vi "Unzip-Mercury-iXX.vi"(8 "error in (no error)":errorcluster) -> (0 "error out":errorcluster)   [LabVIEW 2019]
uses:
  <userlib>/_OpenG.lib/string/string.llb/Trim Whitespace (String)__ogtk.vi
  <vilib>/zip/NI_Unzip.lvlib
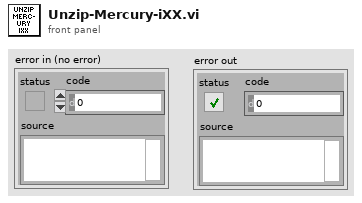
[diagram p1: front panel]
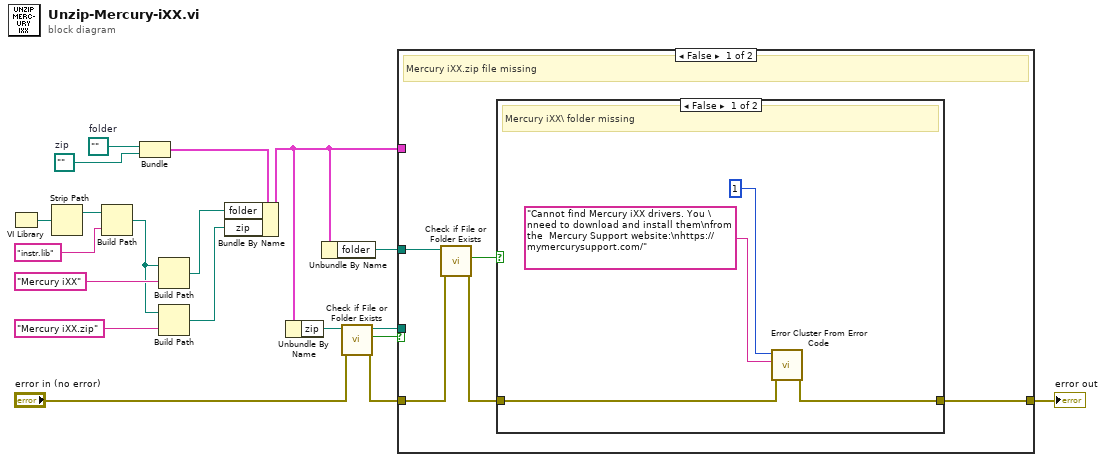
[diagram p0: block diagram]
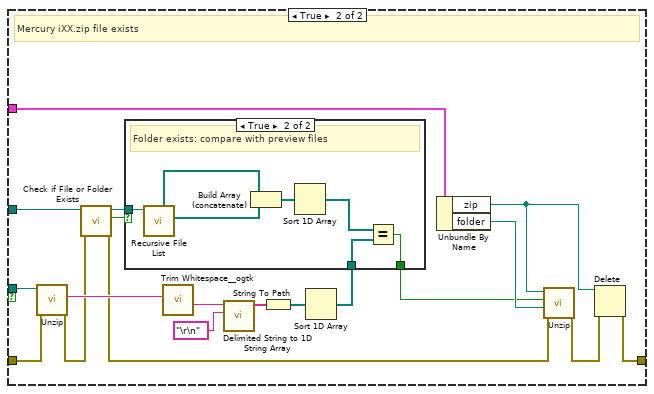
[diagram p3: hidden frame]
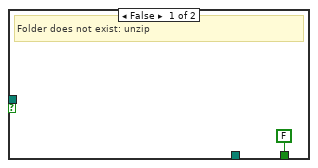
[diagram p4: hidden frame]
diagram:
  w13 = path ""  # zip
  w14 = path ""  # folder
  n1 = VI Library() -> (path=w19:path)
  n2 = Strip Path(path=w19) -> (stripped path=w18:path)  [unwired: 1 out]
  n3 = Build Path(base path=w18, name or relative path="instr.lib") -> (appended path=w15:path)
  n4 = Bundle("folder"=w14, "zip"=w13) -> (w12:cluster{"folder":path, "zip":path})  [unwired: 1 in]
  n5 = Build Path(base path=w15, name or relative path="Mercury iXX") -> (appended path=w11:path)
  n6 = Build Path(base path=w15, name or relative path="Mercury iXX.zip") -> (appended path=w10:path)
  n7 = Bundle By Name(cluster=w12, "folder"=w11, "zip"=w10) -> (w5:cluster{"folder":path, "zip":path})
  n8 = Unbundle By Name(w5) -> ("zip"=w9:path)
  n9 = Unbundle By Name(w5) -> ("folder"=w6:path)
  n10 = call <vilib>:"Check if File or Folder Exists.vi"("error in (no error)"="error in (no error)", "path"=w9) -> ("error out"=w3:errorcluster, "file or folder exists?"=w2:bool, "dup path"=w4:path)  [unwired: 7 in]
  n11 = case shown="False" w2 {
    tunnel: [w20 w48] -> w8
    tunnel: w6 -> [w24 w47]
    tunnel: w5 -> [_ w46]
    tunnel: w4 -> [_ w39]
    tunnel: w3 -> [w23 w37]
    frame False {
      # "Mercury iXX.zip file missing"
      n12 = call <vilib>:"Check if File or Folder Exists.vi"("error in (no error)"=w23, "path"=w24) -> ("error out"=w21:errorcluster, "file or folder exists?"=w22:bool)  [unwired: 7 in, 1 out]
      n13 = case shown="False" w22 {
        tunnel: w21 -> [w28 w29]
        tunnel: [w25 w29] -> w20
        frame False {
          # "Mercury iXX\\ folder missing"
          n14 = call <vilib>:"Error Cluster From Error Code.vi"("error in (no error)"=w28, "error message (\"\")"="Cannot find Mercury iXX drivers. You \nneed to download and install them\nfrom the  Mercury Support website:\nhttps://mymercurysupport.com/" ("message"), "error code (0)"=1) -> ("error out"=w25:errorcluster)  [unwired: 6 in]
        }
        frame True {
          # "validate if contents are ok?"
          # "Mercury iXX\\ folder exists"
        }
      }
    }
    frame True {
      # "Mercury iXX.zip file exists"
      n15 = call <vilib>:"Unzip.vi"("error in (no error)"=w37, "Zip file"=w39) -> ("error out"=w33:errorcluster, "Preview"=w41:string)  [unwired: 7 in, 1 out]
      n16 = call <vilib>:"Check if File or Folder Exists.vi"("error in (no error)"=w33, "path"=w47) -> ("error out"=w32:errorcluster, "file or folder exists?"=w34:bool, "dup path"=w38:path)  [unwired: 7 in]
      n17 = call-poly <userlib>:"Trim Whitespace__ogtk.vi"("String in"=w41) -> ("String out"=w40:string)  [unwired: 6 in]
      n18 = call <vilib>:"Delimited String to 1D String Array.vi"("delimiter"="\r\n", "delimited string"=w40) -> ("string array"=w43:string[])  [unwired: 9 in]
      n19 = String To Path(string=w43) -> (path=w42:path[])
      n20 = Sort 1D Array(array=w42) -> (sorted array=w36:path[])
      n21 = case shown="True" w34 {
        tunnel: w38 -> [_ w53]
        tunnel: w36 -> [_ w52]
        tunnel: [FALSE w51] -> w35
        frame False {
          # "Folder does not exist: unzip"
        }
        frame True {
          # "Folder exists: compare with preview files"
          n22 = call <vilib>:"Recursive File List.vi"("Folder Path"=w53) -> ("All Files in Dir"=w55:path[], "All Folders"=w56:path[])  [unwired: 6 in, 3 out]
          n23 = Build Array (concatenate)(w56, w55) -> (w54:path[])
          n24 = Sort 1D Array(array=w54) -> (sorted array=w50:path[])
          n25 = Equal?(x=w50, y=w52) -> (x = y?=w51:bool)
        }
      }
      n26 = Unbundle By Name(w46) -> ("zip"=w30:path, "folder"=w45:path)
      n27 = call <vilib>:"Unzip.vi"("error in (no error)"=w32, "Target directory (same as Zip file if empty)"=w45, "Preview only?"=w35, "Zip file"=w30) -> ("error out"=w31:errorcluster)  [unwired: 5 in, 2 out]
      n28 = Delete(path (use dialog)=w30, error in=w31) -> (error out=w48:errorcluster)  [unwired: 3 in, 2 out]
    }
  }
  "error out" <- w8
